vi "MathcadPrime2 attempt to control a variable.vi"() -> ()   [LabVIEW 2011]
uses:
  Variable cluster.ctl
panel:
  out "this fails":string
  out "this works":string
  in  "MathcadPrime.IMathcadPrimeApplication2 2":refnum<k7>
  in  "path":path=path "C:/Users/design/Documents/Final Designs/ADT Designs/EtFlocSedFi/junk2.mcdx"
  out "Variable Clusters out":T1
  in  "Save Worksheet":bool
  in  "stop":bool
  in  "value in":dbl
  in  "units in":string
  out "results out":dbl
  out "units out":string
  out "SetValue":i32
  out "Array 4":string[](array[string])
  out "Array 3":dbl[](array[numeric])
  out "Array 2":errorcluster[](array[cluster])
  out "Array":string[](array[string])
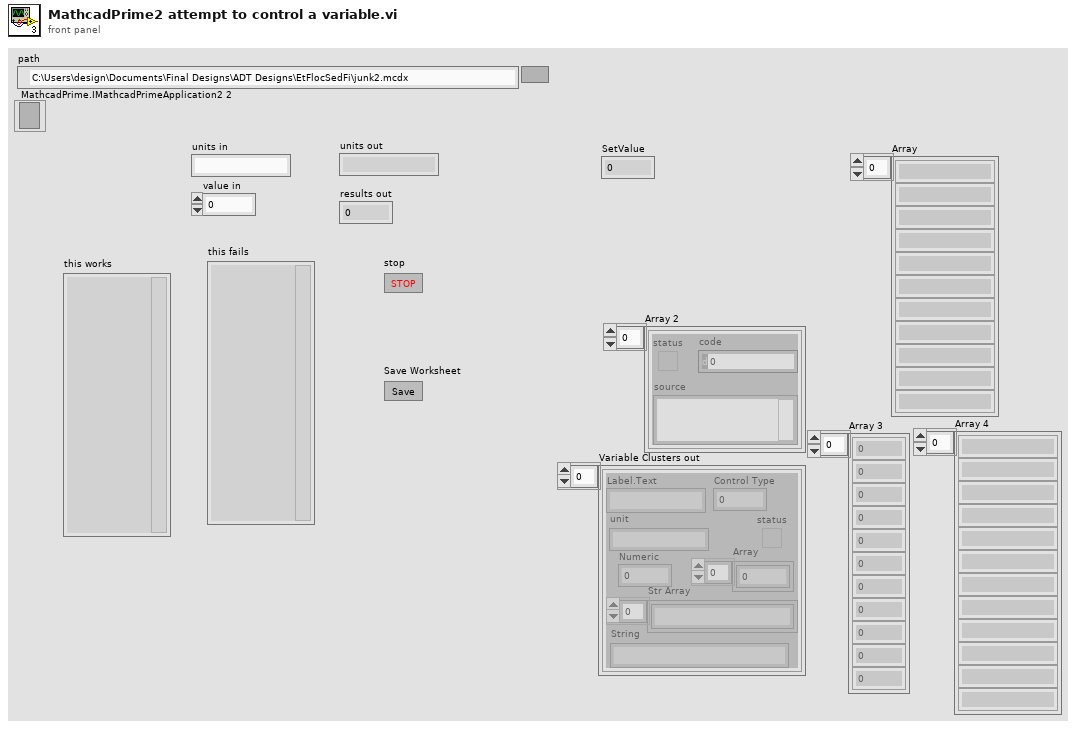
[diagram p1: front panel]
types:
  T1 = typedef "Variable cluster.ctl" = cluster{"Label.Text":string, "Control Type":u32, "Numeric":dbl, "Array":dbl[], "status":bool, "Str Array":string[], "String":string, "unit":string}[]
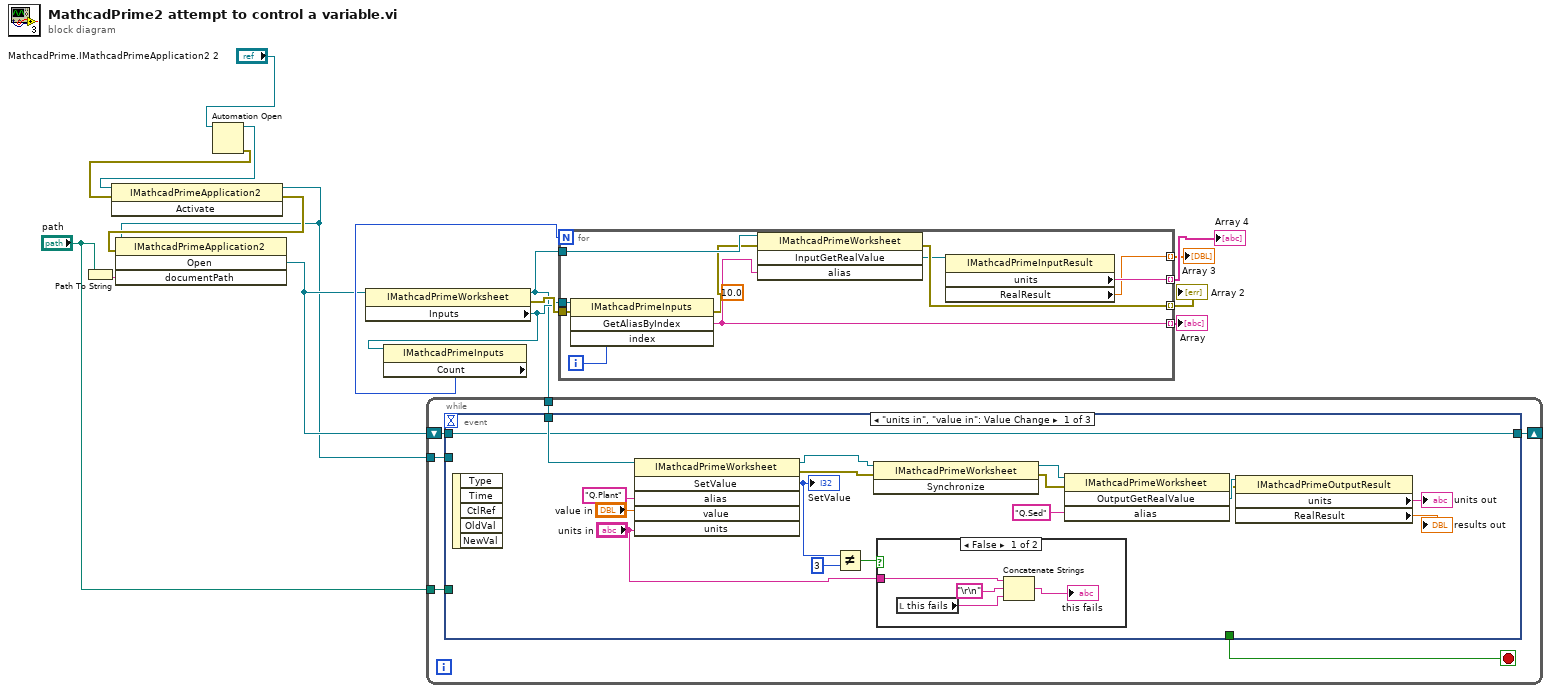
[diagram p0: block diagram]
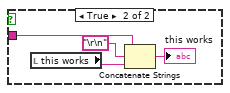
[diagram p2: hidden frame]
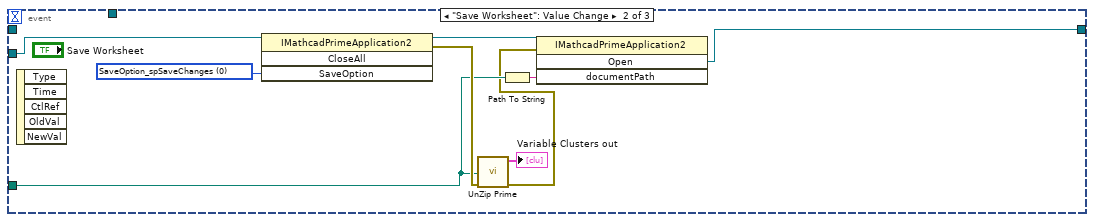
[diagram p3: hidden frame]
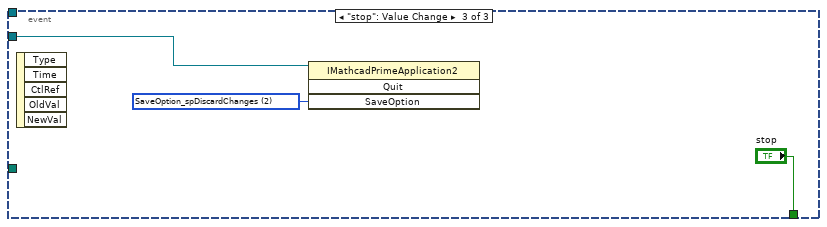
[diagram p4: hidden frame]
diagram:
  n1 = Path To String(path="path") -> (string=w4:string)
  n2 = Automation Open(Automation Refnum="MathcadPrime.IMathcadPrimeApplication2 2") -> (Automation Refnum=w16:refnum<k7>, error out=w14:errorcluster)  [unwired: 3 in]
  n3 = invoke class="IMathcadPrimeApplication2" method="Activate"(reference=w16, error in=w14) -> (reference out=w2:refnum<k7>, error out=w15:errorcluster)  [unwired: 1 in, 1 out]
  n4 = invoke class="IMathcadPrimeApplication2" method="Open"(reference=w2, error in=w15, "documentPath"=w4) -> ("Open"=w5:refnum<k7>)  [unwired: 1 in, 3 out]
  n5 = property class="IMathcadPrimeWorksheet"(reference=w5) -> (reference out=w6:refnum<k7>, error out=w13:errorcluster, "Inputs"=w8:refnum<k7>)  [unwired: 1 in]
  n6 = property class="IMathcadPrimeInputs"(reference=w8) -> ("Count"=w7:i32)  [unwired: 1 in, 2 out]
  n7 = while {
    tunnel: w6 -> [w22]
    tunnel: w2 -> [w19]
    tunnel: "path" -> [w18]
    shift-right: [w17] -> _
    shift-left: w5 -> [w20]
    stop <- w21 stop-if-true
    n8 = event shown="[0] \"units in\", \"value in\": Value Change" {
      selector: _ -> [_ _ _]
      dyn-events: _ -> [_ _ _]
      timeout: _ -> [_ _ _]
      tunnel: w22 -> [w39 _ _]
      tunnel: [_ _ "stop"] -> w21
      tunnel: w20 -> [w29 _ _]
      tunnel: w19 -> [_ w55 w58]
      tunnel: w18 -> [_ w50 _]
      tunnel: [w29 w48 _] -> w17
      event "units in", "value in": Value Change {
        n9 = event-data() -> ()  [unwired: 1 in, 5 out]
        n10 = invoke class="IMathcadPrimeWorksheet" method="SetValue"(reference=w39, "alias"="Q.Plant", "value"="value in", "units"="units in") -> (reference out=w28:refnum<k7>, error out=w26:errorcluster, "SetValue"=w32:i32)  [unwired: 2 in, 3 out]
        "SetValue" <- w32
        n11 = Not Equal?(x=w32, y=3) -> (x != y?=w30:bool)
        n12 = invoke class="IMathcadPrimeWorksheet" method="Synchronize"(reference=w28, error in=w26) -> (reference out=w27:refnum<k7>, error out=w25:errorcluster)  [unwired: 1 in, 1 out]
        n13 = case shown="False" w30 {
          tunnel: "units in" -> [w41 w46]
          frame False {
            n14 = local read "this fails"() -> (w43:string)
            n15 = Concatenate Strings(w41, "\r\n", w43) -> (→"this fails":string)
          }
          frame True {
            n16 = local read "this works"() -> (w47:string)
            n17 = Concatenate Strings(w46, "\r\n", w47) -> (→"this works":string)
          }
        }
        n18 = invoke class="IMathcadPrimeWorksheet" method="OutputGetRealValue"(reference=w27, error in=w25, "alias"="Q.Sed") -> (error out=w24:errorcluster, "OutputGetRealValue"=w36:refnum<k7>)  [unwired: 1 in, 2 out]
        n19 = property class="IMathcadPrimeOutputResult"(reference=w36, error in=w24) -> ("units"=→"units out":string, "RealResult"=→"results out":dbl)  [unwired: 2 out]
      }
      event "Save Worksheet": Value Change {
        w54 = 0 items=["SaveOption_spSaveChanges", "SaveOption_spPromptToSaveChanges", "SaveOption_spDiscardChanges"] ("SaveOption")
        n20 = event-data() -> ()  [unwired: 1 in, 5 out]
        n21 = invoke class="IMathcadPrimeApplication2" method="CloseAll"(reference=w55, "SaveOption"=w54) -> (reference out=w52:refnum<k7>, error out=w53:errorcluster)  [unwired: 2 in, 2 out]
        n22 = call "UnZip Prime.vi"("error in"=w53, "Path"=w50) -> ("error out"=w49:errorcluster, "Variable Clusters out"=→"Variable Clusters out":T1)  [unwired: 8 in]
        n23 = Path To String(path=w50) -> (string=w51:string)
        n24 = invoke class="IMathcadPrimeApplication2" method="Open"(reference=w52, error in=w49, "documentPath"=w51) -> ("Open"=w48:refnum<k7>)  [unwired: 1 in, 3 out]
      }
      event "stop": Value Change {
        w57 = 2 items=["SaveOption_spSaveChanges", "SaveOption_spPromptToSaveChanges", "SaveOption_spDiscardChanges"] ("SaveOption")
        n25 = event-data() -> ()  [unwired: 1 in, 5 out]
        n26 = invoke class="IMathcadPrimeApplication2" method="Quit"(reference=w58, "SaveOption"=w57) -> ()  [unwired: 2 in, 4 out]
      }
    }
  }
  n27 = for {
    N: w7 -> [_]
    tunnel: w13 -> [w69]
    tunnel: w8 -> [w68]
    tunnel: [w66] -> w12 mode=indexing
    tunnel: [w63] -> w11 mode=indexing
    tunnel: w6 -> [w65]
    tunnel: [w61] -> w10 mode=indexing
    tunnel: [w60] -> w9 mode=indexing
    i -> [w67]
    (unwired) 10.0 ("value")
    n28 = invoke class="IMathcadPrimeInputs" method="GetAliasByIndex"(reference=w68, error in=w69, "index"=w67) -> (error out=w64:errorcluster, "GetAliasByIndex"=w66:string)  [unwired: 1 in, 2 out]
    n29 = invoke class="IMathcadPrimeWorksheet" method="InputGetRealValue"(reference=w65, error in=w64, "alias"=w66) -> (error out=w63:errorcluster, "InputGetRealValue"=w62:refnum<k7>)  [unwired: 1 in, 2 out]
    n30 = property class="IMathcadPrimeInputResult"(reference=w62) -> ("units"=w61:string, "RealResult"=w60:dbl)  [unwired: 1 in, 2 out]
  }
  "Array" <- w12
  "Array 2" <- w11
  "Array 3" <- w9
  "Array 4" <- w10
